vi "ArmXZToLE.vi"(9 "Z":dbl, 11 "X":dbl) -> (1 "Extend":dbl, 2 "Lift":dbl)   [LabVIEW 2020]
doc: "Take X, Y and Z values and output, with complicated math, Rotate, Lift, Extend values to get to that point\n\nInputs:\n--X--Double\n--Y--Double\n--Z--Double\n\nOutputs:\n--Rotate--Double--Degrees\n--Lift--Double--Degrees\n--Extend--Double--Inches"
uses:
  <vilib>/Rock Robotics/WPI/ThirdParty/JAS_Junk/TrajLib/Trajectory_Library.lvlib
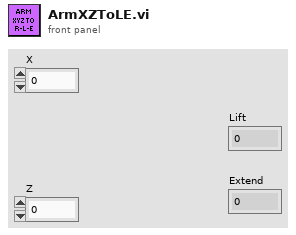
[diagram p1: front panel]
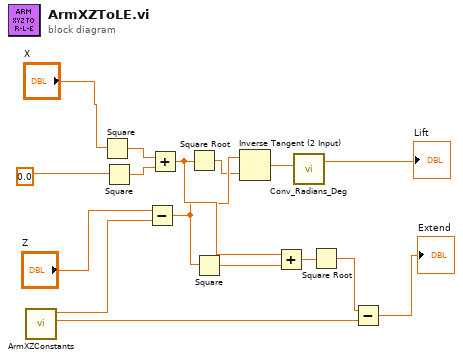
[diagram p0: block diagram]
diagram:
  n1 = call "ArmXZConstants.vi"() -> ("Unextended Length (in)"=w6:dbl, "Pivot Height (in)"=w8:dbl)  [unwired: 10 in]
  n2 = Square(x="X") -> (x^2=w16:dbl)
  n3 = Square(x=0.0) -> (x^2=w15:dbl)
  n4 = Subtract(x="Z", y=w8) -> (x-y=w3:dbl)
  n5 = Add(x=w16, y=w15) -> (x+y=w11:dbl)
  n6 = Square Root(x=w11) -> (sqrt(x)=w2:dbl)
  n7 = Square(x=w3) -> (x^2=w10:dbl)
  n8 = Inverse Tangent (2 Input)(1:w2, 2:w3) -> (0:w13:dbl)
  n9 = Add(x=w11, y=w10) -> (x+y=w9:dbl)
  n10 = call <vilib>:"Conv_Radians_Deg.vi"("Radians"=w13) -> ("Degrees"=→"Lift":dbl)  [unwired: 10 in]
  n11 = Square Root(x=w9) -> (sqrt(x)=w7:dbl)
  n12 = Subtract(x=w7, y=w6) -> (x-y=→"Extend":dbl)
